vi "Launch.vi"(9 "Queue Actor":refnum<class "Queue Actor.lvclass">, 10 "Alias":string) -> (0 "error out":errorcluster)   [LabVIEW 2021, in "jettl Queue Actor.lvlib"]
uses:
  jettl Queue Actor.lvlib
  jettl Queue Actor/jettl Queue Actor.lvclass
  Actor/Queue Actor/Queue Actor.lvclass
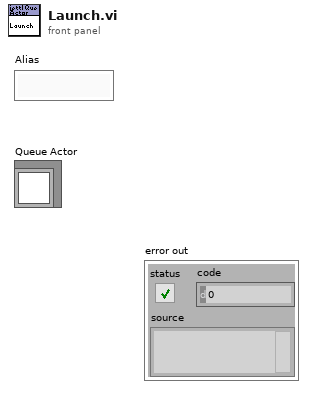
[diagram p1: front panel]
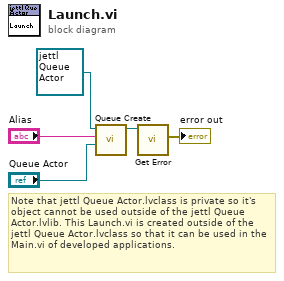
[diagram p0: block diagram]
diagram:
  # "Note that jettl Queue Actor.lvclass is private so it's object cannot be used outside of the jettl Queue Actor.lvlib. This Launch.vi is created outside of the jettl Queue Actor.lvclass so that it can be used in the Main.vi of developed applications."
  n1 = call-dynamic "Queue Create.vi"("Queue Actor"="Queue Actor", "Alias"="Alias", "jettl Queue Actor in"=refnum<class "jettl Queue Actor.lvclass"> refnum ("jettl.lvlib:jettl Queue Actor.lvlib:jettl Queue Actor.lvclass")) -> ("jettl Queue Actor out"=w4:refnum<class "jettl Queue Actor.lvclass">)  [unwired: 8 in]
  n2 = call-dynamic "Get Error.vi"("jettl Queue Actor in"=w4) -> ("Error"=→"error out":errorcluster)  [unwired: 10 in]
